vi "Configure Voltage Edge Time Test.vi"(8 "error in (no error)":errorcluster, 9 "Voltage Fall  (1)":dbl=1.0 min=0.0001 max=500.0 step=1.0 format="%#.4f", 10 "Voltage Rise (1)":dbl=1.0 min=0.0001 max=500.0 step=1.0 format="%#.4f", 11 "VISA resource name":refnum<visa-resource-name>) -> (0 "error out":errorcluster, 3 "VISA resource name out":refnum<visa-resource-name>)   [LabVIEW 2019, in "BK Precision 8500B Series.lvlib"]
doc: "Configures the voltage level to start the Rise (low) or Fall (high) Test. The voltage entered will work as a marker to start the timing of the voltage rise/fall."
uses:
  <instrlib>/BK Precision 8500B Series/BK Precision 8500B Series.lvlib
panel:
  # "V"
  # "V"
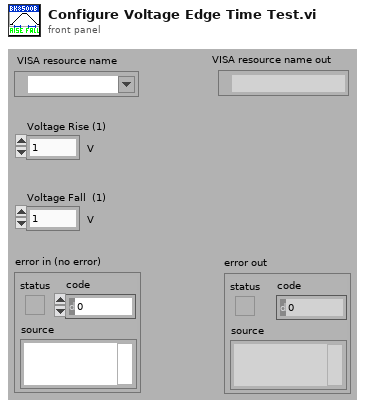
[diagram p1: front panel]
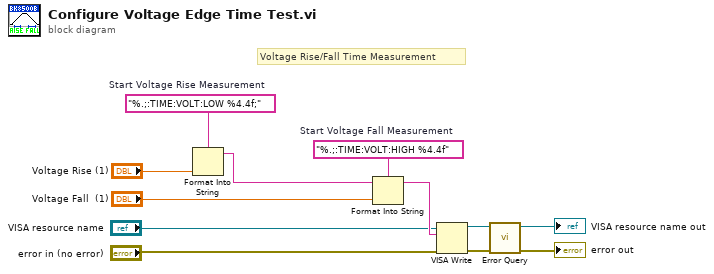
[diagram p0: block diagram]
diagram:
  w5 = "%.;:TIME:VOLT:HIGH %4.4f"  # Start Voltage Fall Measurement
  w8 = "%.;:TIME:VOLT:LOW %4.4f;"  # Start Voltage Rise Measurement
  # "Voltage Rise/Fall Time Measurement"
  n1 = Format Into String(format string=w8, "Voltage Rise (1)") -> (resulting string=w3:string)  [unwired: 2 in, 1 out]
  n2 = Format Into String(format string=w5, initial string=w3, "Voltage Fall  (1)") -> (resulting string=w4:string)  [unwired: 1 in, 1 out]
  n3 = VISA Write(VISA resource name="VISA resource name", write buffer=w4, error in (no error)="error in (no error)") -> (VISA resource name out=w9:refnum<visa-resource-name>, error out=w10:errorcluster)  [unwired: 1 out]
  n4 = call <instrlib>:"Error Query.vi"("error in (no error)"=w10, "VISA resource name"=w9) -> ("error out"=→"error out":errorcluster, "VISA resource name out"=→"VISA resource name out":refnum<visa-resource-name>)  [unwired: 6 in, 2 out]
